vi "Turret Structure.vi"(0 "AIDeviceRef":T1, 1 "Raw Turret":dbl, 2 "upper limit":dbl=4.5, 3 "lower limit":dbl=0.85, 5 "Turret Case":i32, 7 "Home Speed":dbl=1.0, 9 "Home postion":dbl, 11 "error in (no error)":errorcluster) -> (6 "Turret Output":dbl, 15 "Turret Case Output":dbl)   [LabVIEW 2011]
uses:
  <vilib>/Rock Robotics/WPI/AnalogChannel/WPI_AnalogChannelDevRef.ctl
  <vilib>/Rock Robotics/SystemInterfaces/Typedef/FPGA_TypedefAnalogModule.ctl
  <vilib>/Rock Robotics/SystemInterfaces/AI/FPGA_AIChannel.ctl
  <vilib>/addons/control/pid/pid.llb/PID (DBL).vi
  <vilib>/addons/control/pid/NI_PID_pid.lvlib
panel:
  in  "-1/1 per degree":dbl=0.05
  in  "Volts per degree":dbl=0.0166666666666667
  in  "PID Gains":T4={"proportional gain (Kc)"=1.0, "integral time (Ti, min)"=0.01, "derivative time (Td, min)"=0.0} {"derivative time (Td, min)" format="%.3f"; "integral time (Ti, min)" format="%.3f"; "proportional gain (Kc)" format="%.3f"}
  out "Waveform Chart":dynamicdata(graph)
  in  "PID Enable":bool
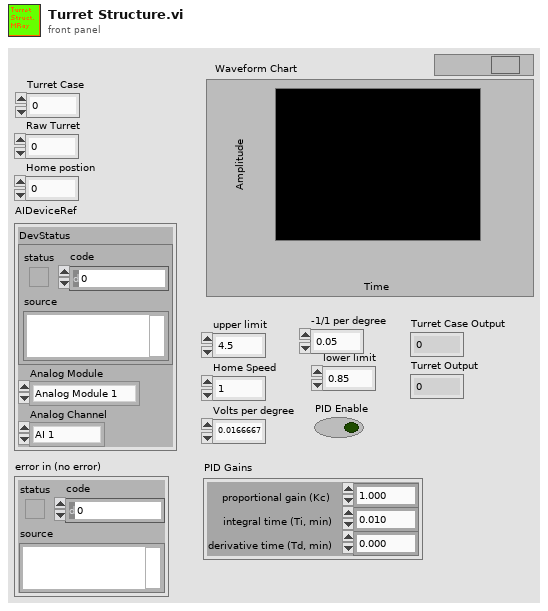
[diagram p1: front panel]
types:
  T1 = typedef "WPI_AnalogChannelDevRef.ctl" = cluster{"DevStatus":errorcluster, "Analog Module":T2, "Analog Channel":T3}
  T2 = typedef "FPGA_TypedefAnalogModule.ctl" = enum16{"Analog Module 1", "Analog Module 2"}
  T3 = typedef "FPGA_AIChannel.ctl" = enum8{"AI 1", "AI 2", "AI 3", "AI 4", "AI 5", "AI 6", "AI 7", "AI 8", "Invalid"}
  T4 = cluster{"proportional gain (Kc)":dbl, "integral time (Ti, min)":dbl, "derivative time (Td, min)":dbl}
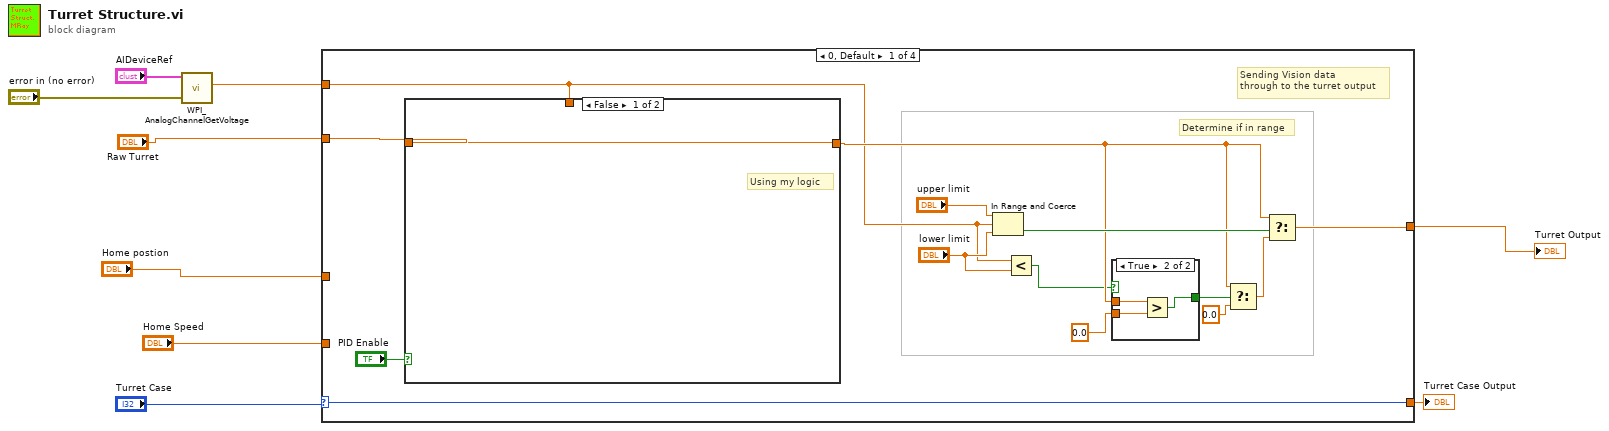
[diagram p0: block diagram]
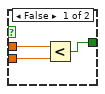
[diagram p2: hidden frame]
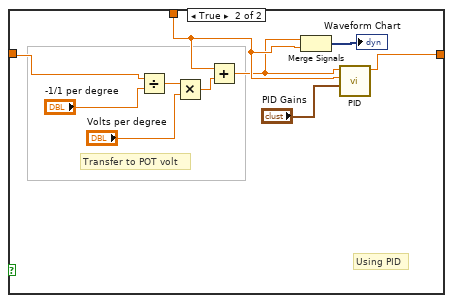
[diagram p3: hidden frame]
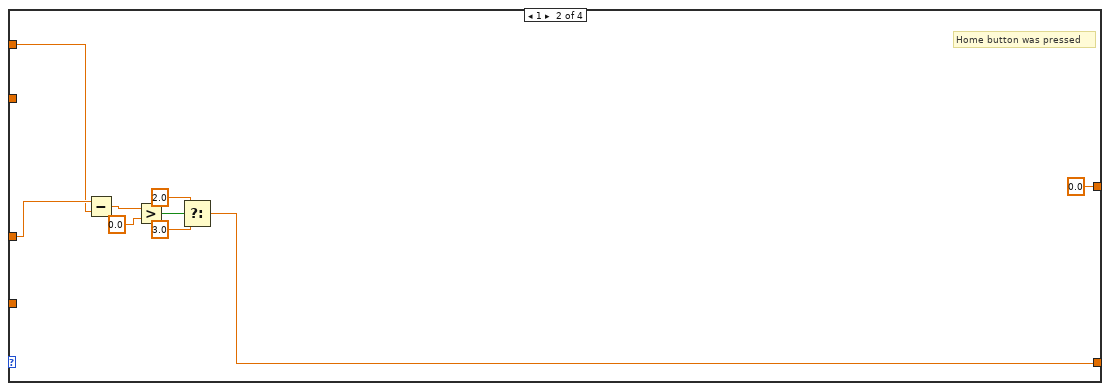
[diagram p4: hidden frame]
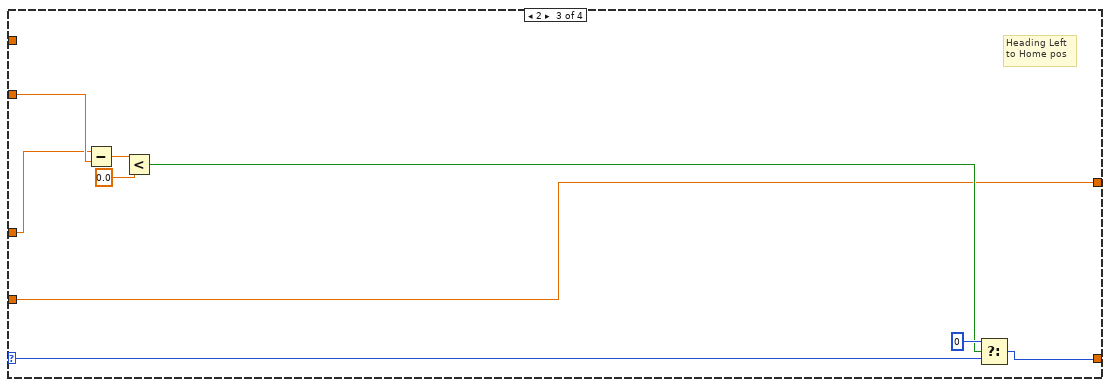
[diagram p5: hidden frame]
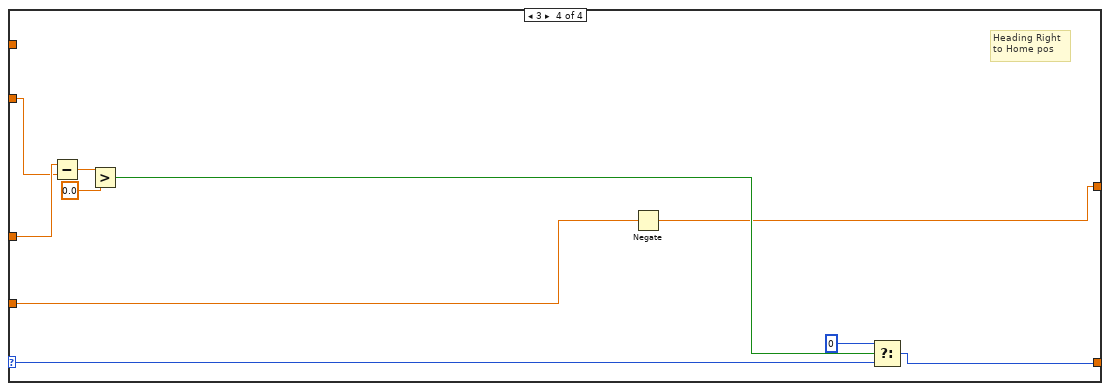
[diagram p6: hidden frame]
diagram:
  n1 = call <vilib>:"WPI_AnalogChannelGetVoltage.vi"("error in (no error)"="error in (no error)", "AIDeviceRef"="AIDeviceRef") -> ("Voltage"=w9:dbl)  [unwired: 7 in, 2 out]
  n2 = case shown="0, Default" "Turret Case" {
    selector: "Turret Case" -> [w12 _ w53 w63]
    tunnel: w9 -> [w11 w43 _ _]
    tunnel: "Raw Turret" -> [w20 _ w56 w65]
    tunnel: [w13 0.0 ("Home Speed 2") w50 w59] -> w8
    tunnel: "Home postion" -> [_ w44 w55 w66]
    tunnel: [w12 w42 w52 w62] -> w1
    tunnel: "Home Speed" -> [_ _ w50 w60]
    frame 0, Default {
      # "Determine if in range"
      # "Sending Vision data\nthrough to the turret output"
      n3 = case shown="False" "PID Enable" {
        tunnel: w20 -> [w30 w39]
        tunnel: [w30 w34] -> w16
        tunnel: w11 -> [_ w32]
        frame False {
          # "Using my logic"
        }
        frame True {
          # "Transfer to POT volt"
          # "Using PID"
          n4 = Divide(x=w39, y="-1/1 per degree") -> (x/y=w38:dbl)
          n5 = Multiply(x=w38, y="Volts per degree") -> (x*y=w36:dbl)
          n6 = Add(x=w32, y=w36) -> (x+y=w31:dbl)
          n7 = Merge Signals(w31, w32) -> (→"Waveform Chart":dynamicdata)
          n8 = call-poly <vilib>:"PID.vi"("PID gains"="PID Gains", "process variable"=w32, "setpoint"=w31) -> ("output"=w34:dbl)  [unwired: 7 in, 1 out]
        }
      }
      n9 = In Range and Coerce(upper limit="upper limit", x=w11, lower limit="lower limit") -> (In Range?=w21:bool)  [unwired: 1 out]
      n10 = Less?(x=w11, y="lower limit") -> (x < y?=w10:bool)
      n11 = case shown="True" w10 {
        tunnel: 0.0 -> [w25 w29]
        tunnel: [w24 w28] -> w17
        tunnel: w16 -> [w26 w27]
        frame False {
          n12 = Less?(x=w26, y=w25) -> (x < y?=w24:bool)
        }
        frame True {
          n13 = Greater?(x=w27, y=w29) -> (0:w28:bool)
        }
      }
      n14 = Select(t=w16, s=w17, f=0.0) -> (s? t:f=w15:dbl)
      n15 = Select(t=w16, s=w21, f=w15) -> (s? t:f=w13:dbl)
    }
    frame 1 {
      # "Home button was pressed"
      n16 = Subtract(x=w44, y=w43) -> (x-y=w45:dbl)
      n17 = Greater?(x=w45, y=0.0) -> (0:w47:bool)
      n18 = Select(t=2.0, s=w47, f=3.0) -> (s? t:f=w42:dbl)
    }
    frame 2 {
      # "Heading Left\nto Home pos"
      n19 = Subtract(x=w55, y=w56) -> (x-y=w57:dbl)
      n20 = Less?(x=w57, y=0.0) -> (x < y?=w51:bool)
      n21 = Select(t=0, s=w51, f=w53) -> (s? t:f=w52:i32)
    }
    frame 3 {
      # "Heading Right\nto Home pos"
      n22 = Subtract(x=w66, y=w65) -> (x-y=w67:dbl)
      n23 = Greater?(x=w67, y=0.0) -> (0:w61:bool)
      n24 = Negate(x=w60) -> (-x=w59:dbl)
      n25 = Select(t=0, s=w61, f=w63) -> (s? t:f=w62:i32)
    }
  }
  "Turret Case Output" <- w1
  "Turret Output" <- w8
